vi "Normalized to Scored.vi"(8 "Penalty":dbl=10.0, 9 "Score":dbl=20.0, 11 "Normalized in":dbl) -> (3 "Score out":dbl)   [LabVIEW 2015]
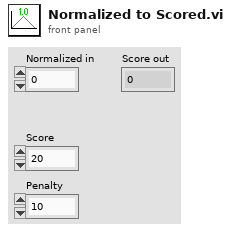
[diagram p1: front panel]
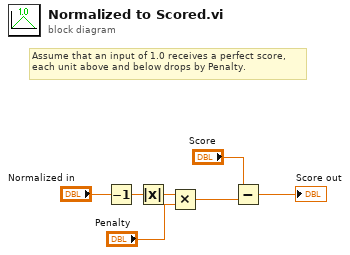
[diagram p0: block diagram]
diagram:
  # "Assume that an input of 1.0 receives a perfect score,\neach unit above and below drops by Penalty."
  n1 = Decrement(x="Normalized in") -> (x-1=w5:dbl)
  n2 = Absolute Value(x=w5) -> (abs(x)=w4:dbl)
  n3 = Multiply(x=w4, y="Penalty") -> (x*y=w3:dbl)
  n4 = Subtract(x="Score", y=w3) -> (x-y=→"Score out":dbl)
